vi "Example2.vi"() -> ()   [LabVIEW 2014, in "Nephelometer.lvclass"]
uses:
  Nephelometer.lvclass
  Reusable/Session APIs/File Access/Config Data/Config Data.lvclass
  Reusable/Session APIs/File Access/Config Data/Config Session.ctl
  <userlib>/_Session Fwk/Session - Root.lvclass
  Reusable/Session APIs/Serial/Serial Session.lvclass
  <vilib>/Platform/TimedLoop/XDataNode/XDataNode.xnode
  <vilib>/Platform/TimedLoop/XDataNode/nitl_modes.ctl
  <vilib>/Platform/TimedLoop/XDataNode/XDNodeRunTimeDep.lvlib
  <vilib>/Platform/TimedLoop/XDataNode/wakeup.ctl
  <vilib>/Platform/TimedLoop/XDataNode/timing_clust.ctl
panel:
  out "error out":errorcluster
  out "Read - Asynchronous":string
  in  "Read":bool
  in  "Boolean":bool
  in  "Write - Asynchronous":string
  in  "cmd":bool
  out "error out 5":errorcluster
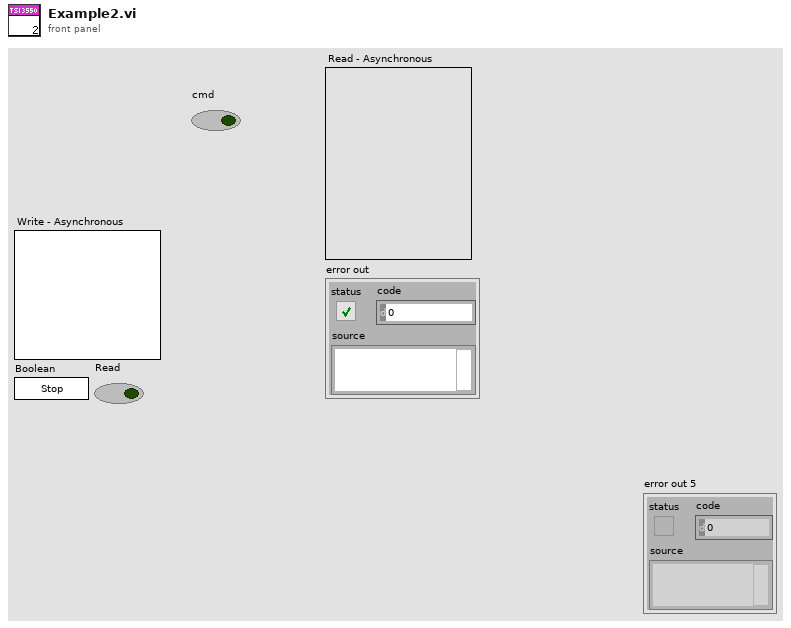
[diagram p1: front panel]
types:
  T1 = typedef "Config Data.lvclass/Config Session.ctl" = refnum<data-value>
  T2 = typedef "Session - Root.lvclass/Session Handle.ctl" = refnum<data-value>
  T3 = typedef "XDNodeRunTimeDep.lvlib/timing_clust.ctl" = cluster{"Expected End [f-1]":u64, "Actual End [f-1]":u64, "Finished Late? [f-1]":bool, "Expected End [i-1]":u64, "Actual End [i-1]":u64, "Finished Late? [i-1]":bool, "Expected Start [i]":u64, "Actual Start [i]":u64, "Expected Start [f]":u64, "Actual Start [f]":u64, "Source Name":string, "Structure Name":string, "Period":i64, "Deadline":i64, "Offset":i64, "Start":i64, "Priority":i32, "Timeout":i32, "Mode":T4, "Wakeup Reason":T5, "Error":errorcluster, "Source Type":string, "Secondary Source Type":string, "Global End Time":u64, "Global Start Time":u64, "Frame Duration":u64, "Iteration Duration":u64, "Assigned CPU":i32, "I/O Scan Engine Mode":u32}
  T4 = typedef "XDNodeRunTimeDep.lvlib/nitl_modes.ctl" = enum32{"No Change", "Process missed periods, maintain original phase", "Discard missed periods, maintain original phase", "Process missed periods, ignore original phase", "Discard missed periods, ignore original phase"}
  T5 = typedef "XDNodeRunTimeDep.lvlib/wakeup.ctl" = enum32{"Normal", "Aborted", "Asynchronous wakeup", "Timing source error", "Timed loop error", "Timeout"}
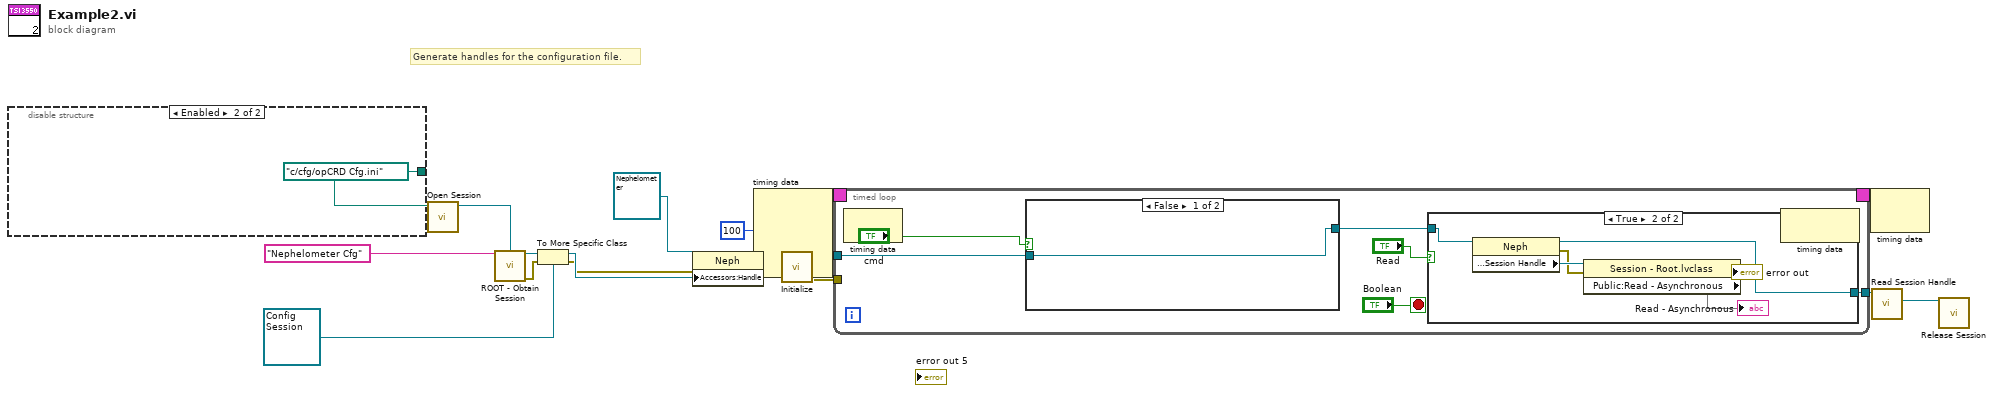
[diagram p0: block diagram]
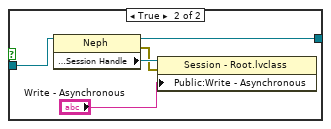
[diagram p3: hidden frame]
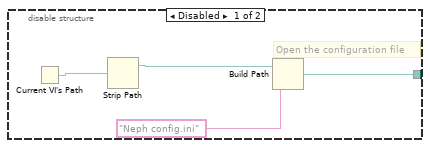
[diagram p4: hidden frame]
diagram:
  # "Generate handles for the configuration file."
  n1 = disable-structure shown="Enabled" {
    disable-tunnel: [w19 path "c:/cfg/opCRD Cfg.ini" ("Path")] -> w15
    frame Disabled {
      # "Open the configuration file"
      n2 = Current VI's Path() -> (path=w22:path)
      n3 = Strip Path(path=w22) -> (stripped path=w21:path)  [unwired: 1 out]
      n4 = Build Path(base path=w21, name or relative path="Neph config.ini") -> (appended path=w19:path)
    }
    frame Enabled {
    }
  }
  n5 = call "Open Session.vi"("Path"=w15) -> ("Config Data"=w18:refnum<class "Config Data.lvclass">)  [unwired: 9 in, 1 out]
  n6 = call <userlib>:"ROOT - Obtain Session.vi"("Session Name ()"="Nephelometer Cfg", "OBJ - Session"=w18) -> ("Session Handle"=w14:T2, "error out"=w13:errorcluster)  [unwired: 11 in, 1 out]
  n7 = To More Specific Class(target class=T1 refnum ("Session Handle"), reference=w14, error in=w13) -> (specific class reference=w11:T1, error out=w10:errorcluster)
  n8 = property class="Neph"(reference=refnum<class "Nephelometer.lvclass"> refnum ("Neph"), error in=w10, "Accessors:Handle"=w11) -> (reference out=w9:refnum<class "Nephelometer.lvclass">, error out=w8:errorcluster)
  n9 = node-c288(i64 100 ("Period")) -> (w3:T3)  [unwired: 3 in]
  n10 = call "Initialize.vi"("error in"=w8, "Neph In"=w9) -> ("error out"=w6:errorcluster, "Neph Out"=w7:refnum<class "Nephelometer.lvclass">)  [unwired: 8 in]
  n11 = timed-loop {
    tunnel: w7 -> [w26]
    tunnel: w6 -> [_]
    tunnel: [w24] -> w4
    timing: w3 -> [_]
    timing-out: [_] -> w2
    stop <- "Boolean" stop-if-true
    n12 = node-c288() -> ()  [unwired: 1 in, 1 out]
    n13 = case shown="False" "cmd" {
      tunnel: w26 -> [w39 w41]
      tunnel: [w39 w40] -> w25
      frame False {
      }
      frame True {
        n14 = property class="Neph"(reference=w41) -> (reference out=w40:refnum<class "Nephelometer.lvclass">, error out=w43:errorcluster, "Accessors:Session Handle"=w44:T2)  [unwired: 1 in]
        n15 = property class="Session - Root.lvclass"(reference=w44, error in=w43, "Public:Write - Asynchronous"="Write - Asynchronous") -> ()  [unwired: 2 out]
      }
    }
    n16 = case shown="True" "Read" {
      tunnel: w25 -> [w32 w35]
      tunnel: [w32 w34] -> w24
      frame False {
      }
      frame True {
        n17 = property class="Neph"(reference=w35) -> (reference out=w34:refnum<class "Nephelometer.lvclass">, error out=w37:errorcluster, "Accessors:Session Handle"=w38:T2)  [unwired: 1 in]
        n18 = property class="Session - Root.lvclass"(reference=w38, error in=w37) -> (error out=→"error out":errorcluster, "Public:Read - Asynchronous"=→"Read - Asynchronous")  [unwired: 1 out]
      }
    }
    n19 = node-c288() -> ()  [unwired: 1 in, 1 out]
  }
  n20 = node-c288(w2) -> ()  [unwired: 1 out]
  n21 = call "Read Session Handle.vi"("Nephelometer in"=w4) -> ("Session Handle"=w5:T2)  [unwired: 8 in, 2 out]
  n22 = call "Release Session.vi"("Session Handle"=w5) -> ()  [unwired: 14 in, 1 out]
